vi "CLC_SA_SignalSYC.vi"(5 "Polarity":u16, 7 "CH_ON/OFF":u16, 10 "Mode":u16, 11 "TCPIPin":T1={"address"="192.168.100.111", "remote port or service name"=5025, "timeout ms (60000)"=10000}) -> (3 "TCPIPout":T1={"address"="192.168.100.111", "remote port or service name"=5025, "timeout ms (60000)"=10000})   [LabVIEW 2023]
panel:
  out "error out":errorcluster
  in  "error in":errorcluster
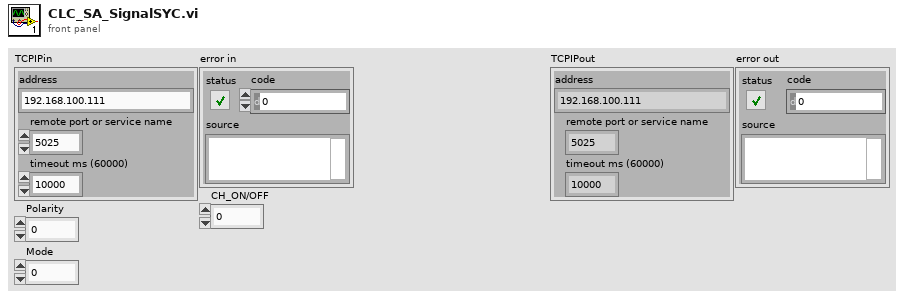
[diagram p1: front panel]
types:
  T1 = cluster{"address":string, "remote port or service name":u16, "timeout ms (60000)":i32}
  T2 = cluster{"Mode":u16, "Polarity":u16, "CH_ON/OFF":u16, "Channel":i32, "Gain":i32, "Phase":i32}
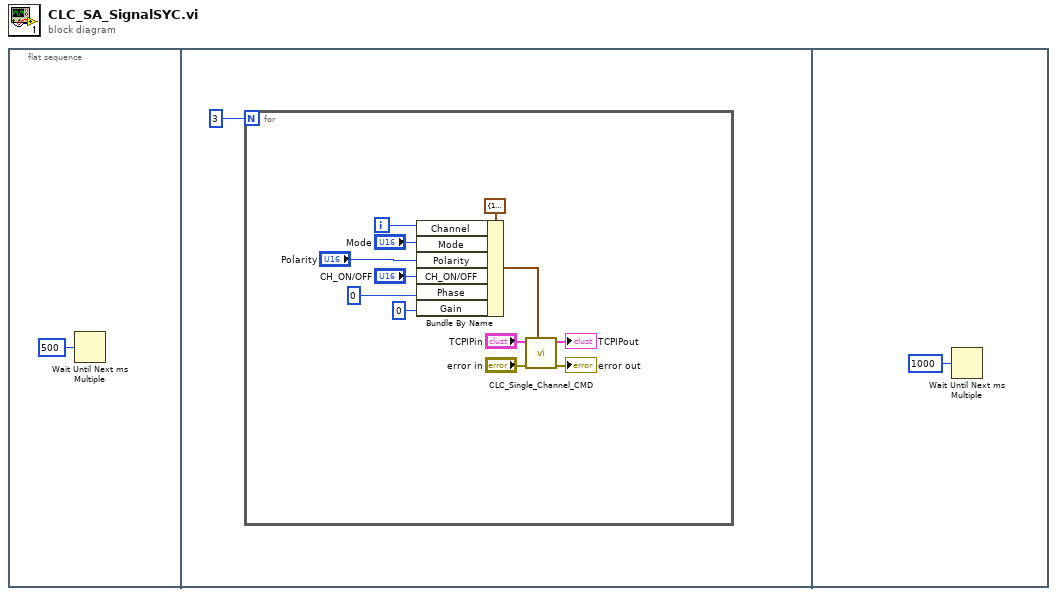
[diagram p0: block diagram]
diagram:
  n1 = flat-sequence {
    frame #0 {
      n2 = Wait Until Next ms Multiple(millisecond multiple=u32 500) -> ()  [unwired: 1 out]
    }
    frame #1 {
      n3 = for {
        N: 3 -> [_]
        i -> [w8]
        n4 = Bundle By Name(cluster=T2 {"Mode"=1, "Polarity"=1, "CH_ON/OFF"=1, "Channel"=0, "Gain"=0, "Phase"=0} ("Channel params"), "Channel"=w8, "Mode"="Mode", "Polarity"="Polarity", "CH_ON/OFF"="CH_ON/OFF", "Phase"=0, "Gain"=0) -> (w13:T2)
        n5 = call "CLC_Single_Channel_CMD.vi"("Channel params"=w13, "error in"="error in", "TCPIPin"="TCPIPin") -> ("error out"=→"error out":errorcluster, "TCPIPout"=→"TCPIPout":T1)  [unwired: 6 in, 1 out]
      }
    }
    frame #2 {
      n6 = Wait Until Next ms Multiple(millisecond multiple=u32 1000) -> ()  [unwired: 1 out]
    }
  }
